vi "Anritsu VNA Read Number of Points.vi"(6 "Channel":i8=1 min=1 max=99 step=1, 7 "Anritsu VNA":T1, 8 "error in (no error)":errorcluster, 11 "VISA Resource Name":refnum<visa-resource-name>) -> (0 "error out":errorcluster, 2 "Number Points":i32, 3 "dup VISA Resource Name":refnum<visa-resource-name>)   [LabVIEW 2011]
doc: "This VI for the HP 8753B is used to read the number of stimulus points."
uses:
  TypeDefs/Anritsu VNA Instrument Info.ctl
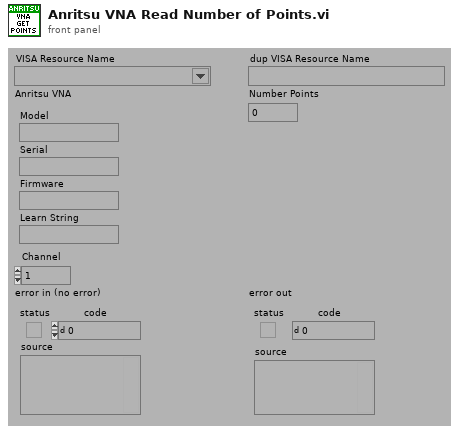
[diagram p1: front panel]
types:
  T1 = typedef "Anritsu VNA Instrument Info.ctl" = cluster{"Model":string, "Serial":string, "Firmware":string, "Learn String":string}
  T2 = typedef "Anritsu VNA Model.ctl" = enum16{"Not Supported", "37XXXX", "MS20XXX", "MS462XX", "MS464XX"}
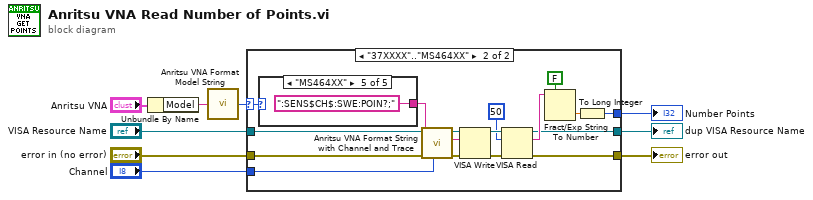
[diagram p0: block diagram]
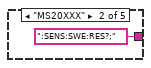
[diagram p4: hidden frame]
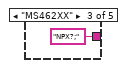
[diagram p5: hidden frame]
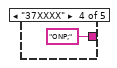
[diagram p6: hidden frame]
diagram:
  n1 = Unbundle By Name("Anritsu VNA") -> ("Model"=w3:string)
  n2 = call "Anritsu VNA Format Model String.vi"("Model"=w3) -> ("Model"=w2:T2)
  n3 = case shown="\"37XXXX\"..\"MS464XX\"" w2 {
    selector: w2 -> [_ w15]
    tunnel: [w11 w23] -> w9
    tunnel: [w10 w22] -> w8
    tunnel: "VISA Resource Name" -> [w11 w21]
    tunnel: "error in (no error)" -> [w10 w20]
    tunnel: [_ w19] -> w5
    tunnel: "Channel" -> [_ w12]
    frame "Not Supported" {
    }
    frame "37XXXX".."MS464XX" {
      n4 = case shown="\"MS464XX\"" w15 {
        tunnel: [_ ":SENS:SWE:RES?;" "NPX?;" "ONP;" ":SENS$CH$:SWE:POIN?;"] -> w14
        frame "Not Supported" {
        }
        frame "MS20XXX" {
        }
        frame "MS462XX" {
        }
        frame "37XXXX" {
        }
        frame "MS464XX" {
        }
      }
      n5 = call "Anritsu VNA Format String with Channel and Trace.vi"("Channel"=w12, "String"=w14) -> ("String Out"=w13:string)  [unwired: 1 in, 6 out]
      n6 = VISA Write(VISA resource name=w21, write buffer=w13, error in (no error)=w20) -> (VISA resource name out=w18:refnum<visa-resource-name>, error out=w26:errorcluster)  [unwired: 1 out]
      n7 = VISA Read(VISA resource name=w18, byte count=u32 50, error in (no error)=w26) -> (VISA resource name out=w23:refnum<visa-resource-name>, read buffer=w25:string, error out=w22:errorcluster)  [unwired: 1 out]
      n8 = Fract/Exp String To Number(use system decimal point (T)=FALSE, string=w25) -> (number=w24:dbl)  [unwired: 3 out]
      n9 = To Long Integer(number=w24) -> (32bit integer=w19:i32)
    }
  }
  "Number Points" <- w5
  "dup VISA Resource Name" <- w9
  "error out" <- w8
